vi "Generate Error.vi"(5 "error code in":i32, 7 "error in":errorcluster, 8 "lv_proc.dll path in":path) -> (0 "error out":errorcluster, 1 "lv_proc.dll path out":path)   [LabVIEW 2013, in "LV Process library.lvlib"]
doc: "Calls lv_proc.dll to convert errors emerged in dll into labview error.\n\nThis vi is intended to use only inside of the LV Process library.\n\n---\nLV Process works only with lv_proc.dll library, which is part of vipm package or should be delivered together with packed library. Placement of this dll is selected in terminal of Create Process.vi."
uses:
  LV Process library.lvlib
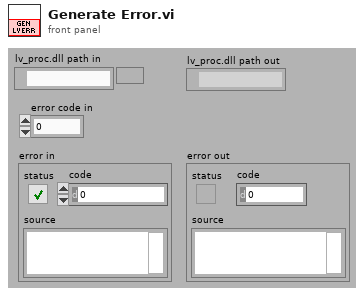
[diagram p1: front panel]
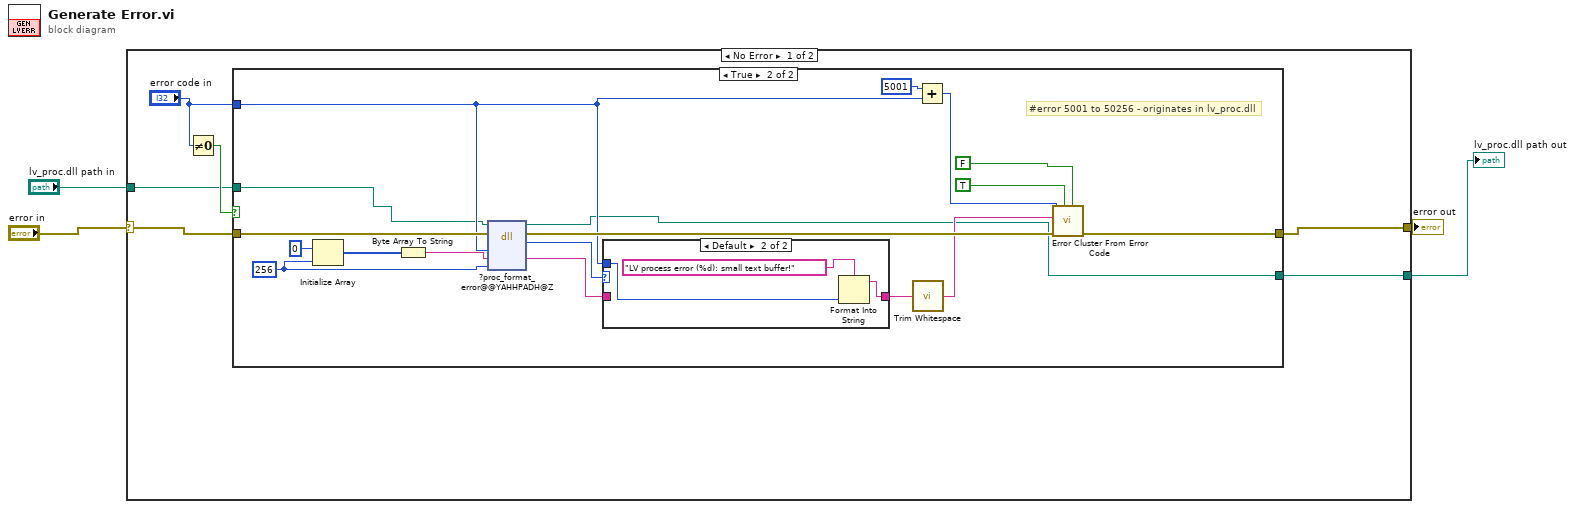
[diagram p0: block diagram]
diagram:
  n1 = case shown="No Error" "error in" {
    selector: "error in" -> [w10 w36]
    tunnel: [w9 w36] -> w3
    tunnel: "lv_proc.dll path in" -> [w6 w35]
    tunnel: [w5 w35] -> w1
    frame No Error {
      n2 = Not Equal To 0?(x="error code in") -> (x != 0?=w7:bool)
      n3 = case shown="True" w7 {
        tunnel: w10 -> [w12 w23]
        tunnel: [w12 w17] -> w9
        tunnel: "error code in" -> [_ w15]
        tunnel: w6 -> [w11 w14]
        tunnel: [w11 w13] -> w5
        frame False {
        }
        frame True {
          w27 = 256 ("dimension size")
          # "#error 5001 to 50256 - originates in lv_proc.dll"
          n4 = Initialize Array(u8 0 ("element"), w27) -> (w30:u8[])
          n5 = Byte Array To String(unsigned byte array=w30) -> (string=w29:string)
          n6 = dll-call lib="C:/Data/GOLPI/LV Process/lv_proc.dll" fn="?proc_format_error@@YAHHPADH@Z" label="proc_format_error"(path in=w14, error in=w23, "code"=w15, "buffer"=w29, "len"=w27) -> (path out=w13:path, error out=w18:errorcluster, "error"=w26:i32, "buffer"=w25:string)  [unwired: 3 in]
          n7 = case shown="Default" w26 {
            tunnel: w25 -> [w31 _]
            tunnel: w15 -> [_ w34]
            tunnel: [w31 w32] -> w24
            frame 0 {
            }
            frame Default {
              n8 = Format Into String(format string="LV process error (%d): small text buffer!", w34) -> (resulting string=w32:string)  [unwired: 2 in, 1 out]
            }
          }
          n9 = call <vilib>:"Trim Whitespace.vi"("string"=w24) -> ("trimmed string"=w16:string)  [unwired: 1 in]
          n10 = Add(x=5001 ("error code (0)"), y=w15) -> (x+y=w19:i32)
          n11 = call <vilib>:"Error Cluster From Error Code.vi"("is warning? (False)"=FALSE, "show call chain? (False)"=TRUE, "error in (no error)"=w18, "error message (\"\")"=w16, "error code (0)"=w19) -> ("error out"=w17:errorcluster)  [unwired: 4 in]
        }
      }
    }
    frame Error {
    }
  }
  "error out" <- w3
  "lv_proc.dll path out" <- w1
